vi "acc and mag WITH multiple file inputs.vi"() -> ()   [LabVIEW 2021]
uses:
  <vilib>/Analysis/baseanly.llb/Mean (DBL).vi
  <vilib>/Utility/file.llb/Read Delimited Spreadsheet (I64).vi
  <vilib>/Analysis/NI_AALBase.lvlib
panel:
  in  "File path":path
  in  "Ending file number":dbl
  in  "Starting file number":dbl
  out "Magnitude vs Time":dbl[][](graph)
  out "subarray":i64[][](array[numeric])
  out "all rows":i64[][](array[numeric])
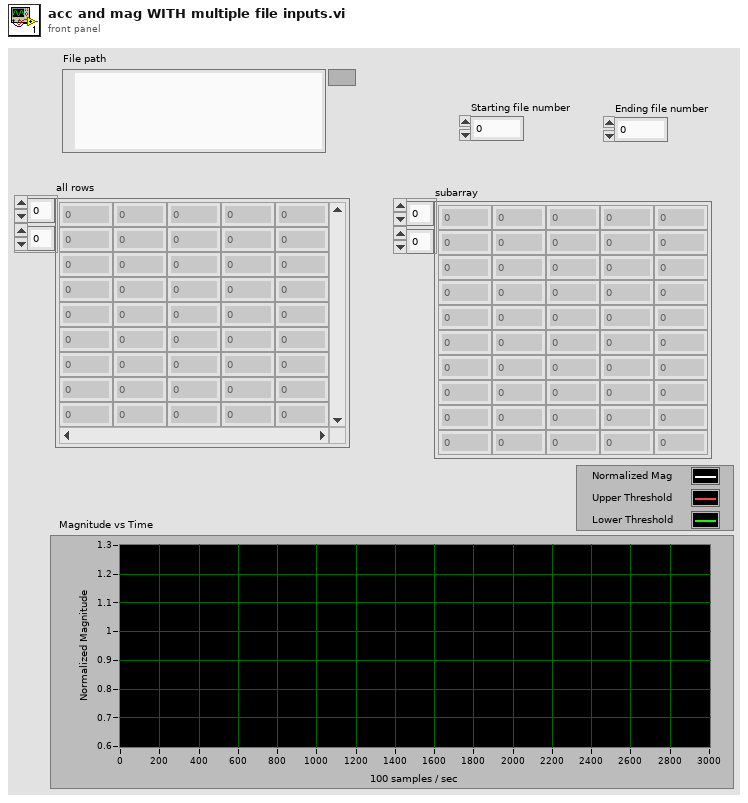
[diagram p1: front panel]
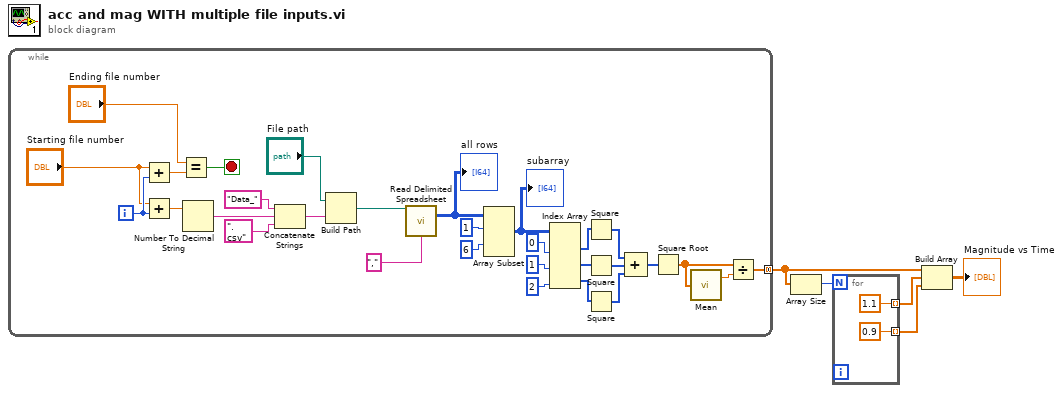
[diagram p0: block diagram]
diagram:
  n1 = while {
    tunnel: [w6] -> w2 mode=concatenating
    i -> [w27]
    stop <- w28 stop-if-true
    n2 = Add(x="Starting file number", y=w27) -> (x+y=w29:dbl)
    n3 = Add(x="Starting file number", y=w27) -> (x+y=w30:dbl)
    n4 = Equal?(x="Ending file number", y=w29) -> (x = y?=w28:bool)
    n5 = Number To Decimal String(number=w30) -> (decimal integer string=w32:string)  [unwired: 1 in]
    n6 = Concatenate Strings("Data_" ("string"), w32, ".csv" ("string")) -> (w34:string)
    n7 = Build Path(base path="File path", name or relative path=w34) -> (appended path=w8:path)
    n8 = call-poly <vilib>:"Read Delimited Spreadsheet.vi"("file path (dialog if empty)"=w8, "delimiter (\\t)"="," ("delimiter (\\t)")) -> ("all rows"=w14:i64[][])  [unwired: 8 in, 5 out]
    "all rows" <- w14
    n9 = Array Subset(array=w14, index (row)=1 ("index"), index (col)=6 ("index")) -> (w15:i64[][])  [unwired: 2 in]
    "subarray" <- w15
    n10 = Index Array(array=w15, index (col) #1=0 ("index (row)"), index (col) #2=1 ("index (row)"), index (col) #3=2 ("disabled index (col)")) -> (element #1=w16:i64[], element #2=w17:i64[], element #3=w18:i64[])  [unwired: 3 in]
    n11 = Square(x=w16) -> (x^2=w19:i64[])
    n12 = Square(x=w17) -> (x^2=w20:i64[])
    n13 = Square(x=w18) -> (x^2=w21:i64[])
    n14 = Compound Arithmetic op=ADD(w19, w20, w21) -> (w22:i64[])
    n15 = Square Root(x=w22) -> (sqrt(x)=w23:dbl[])
    n16 = call-poly <vilib>:"Mean.vi"("X"=w23) -> ("mean"=w24:dbl)  [unwired: 1 out]
    n17 = Divide(x=w23, y=w24) -> (x/y=w6:dbl[])
  }
  n18 = Array Size(array=w2) -> (size(s)=w1:i32)
  n19 = for {
    N: w1 -> [_]
    tunnel: [0.9] -> w4 mode=indexing
    tunnel: [1.1] -> w3 mode=indexing
  }
  n20 = Build Array(w2, w3, w4) -> (→"Magnitude vs Time":dbl[][])
